vi "RDS Check Subscriber.vi"(8 "error in (no error)":errorcluster, 10 "RDS Message In":refnum<class "RDS Message.lvclass">, 11 "RDS Router Subscription in":refnum<class "RDS Router Subscription.lvclass">) -> (0 "error out":errorcluster, 1 "Subscribed?":bool, 2 "RDS Message out":refnum<class "RDS Message.lvclass">, 3 "RDS Child Enqueuer":refnum<class "Message Enqueuer.lvclass">)   [LabVIEW 2015, in "RDS Abstracts.lvlib" / "RDS Router Actor.lvlib" / "RDS Router Subscription.lvclass"]
uses:
  RDS Router Subscription.lvclass
  Libraries/RDS Framework/RDS Message Class/RDS Message.lvclass
  <vilib>/ActorFramework/Message Enqueuer/Message Enqueuer.lvclass
  RDS Router Subscription.lvclass/RDS Router Subscription.ctl
  Libraries/RDS Framework/RDS Message Class/RDS Message.lvclass/RDS Message.ctl
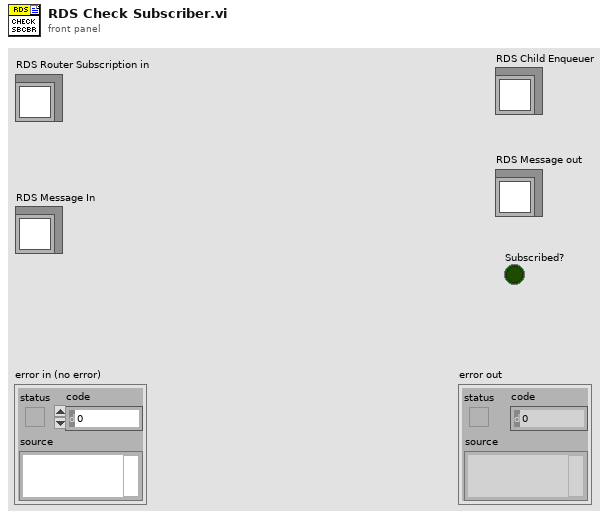
[diagram p1: front panel]
types:
  T1 = typedef "RDS Child Messages.lvlib/RDS Message ID.ctl" = enum16{"RDS Hello World", "String Message", "AIP_Status", "AIP_Command", "GPS_Data", "MCB_Command", "MCB_Status", "Compass_Data", "Depth_Data", "Battery_Data", "Contoller_State", "Set_Mag_Dev", "BTB_Shutdown", "State_Sample_Request", "State_Sample", "PID_Gains_Set", "Helm_Limiter_Set", "Helm_Heading_Command", "Helm_Steering_Command", "Helm_Status", "Controller_Message", "AIP_Set_Min_Depth", "Mission_Controller_State", "Mission_Upload", "Mission_Set_Op_and_Run", "Mission_Settings_Set"}
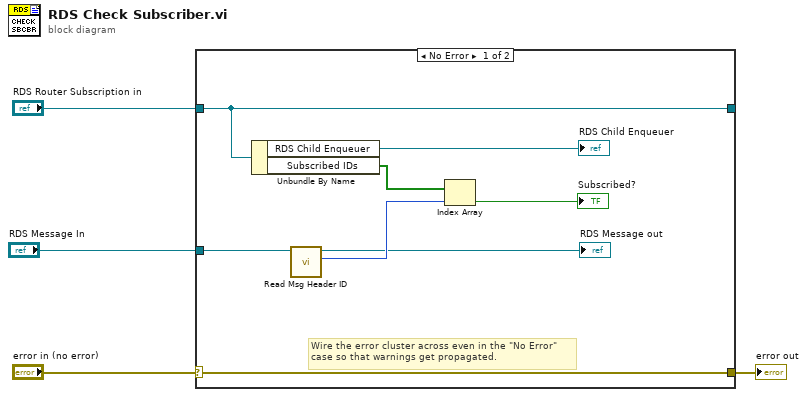
[diagram p0: block diagram]
diagram:
  n1 = case shown="No Error" "error in (no error)" {
    selector: "error in (no error)" -> [w12 w14]
    tunnel: [w12 w14] -> w3
    tunnel: [w11 w13] -> _
    tunnel: "RDS Router Subscription in" -> [w11 w13]
    tunnel: "RDS Message In" -> [w9 _]
    frame No Error {
      # "Wire the error cluster across even in the \"No Error\"\ncase so that warnings get propagated."
      n2 = Unbundle By Name(w11) -> ("RDS Child Enqueuer"=→"RDS Child Enqueuer":refnum<class "Message Enqueuer.lvclass">, "Subscribed IDs"=w8:bool[])
      n3 = call "Read Msg Header ID.vi"("RDS Message in"=w9) -> ("Msg ID"=w7:T1, "RDS Message out"=→"RDS Message out":refnum<class "RDS Message.lvclass">)  [unwired: 6 in, 3 out]
      n4 = Index Array(array=w8, index=w7) -> (element=→"Subscribed?":bool)
    }
    frame Error {
    }
  }
  "error out" <- w3
